vi "FipsAdjacent.vi"() -> (11 "Fips":i32[](array[numeric]))   [LabVIEW 2017] (continued)
VA\"\t51095\n\"New Kent County, VA\"\t51127\t\"King and Queen County, VA\"\t51097\n\"New Kent County, VA\"\t51127\t\"King William County, VA\"\t51101\n\"New Kent County, VA\"\t51127\t\"New Kent County, VA\"\t51127\n\"Northampton County, VA\"\t51131\t\"Accomack County, VA\"\t51001\n\"Northampton County, VA\"\t51131\t\"Mathews County, VA\"\t51115\n\"Northampton County, VA\"\t51131\t\"Middlesex County, VA\"\t51119\n\"Northampton County, VA\"\t51131\t\"Northampton County, VA\"\t51131\n\"Northampton County, VA\"\t51131\t\"York County, VA\"\t51199\n\"Northampton County, VA\"\t51131\t\"Hampton city, VA\"\t51650\n\"Northampton County, VA\"\t51131\t\"Norfolk city, VA\"\t51710\n\"Northampton County, VA\"\t51131\t\"Poquoson city, VA\"\t51735\n\"Northampton County, VA\"\t51131\t\"Virginia Beach city, VA\"\t51810\n\"Northumberland County, VA\"\t51133\t\"St. Mary's County, MD\"\t24037\n\"Northumberland County, VA\"\t51133\t\"Somerset County, MD\"\t24039\n\"Northumberland County, VA\"\t51133\t\"Accomack County, VA\"\t51001\n\"Northumberland County, VA\"\t51133\t\"Lancaster County, VA\"\t51103\n\"Northumberland County, VA\"\t51133\t\"Northumberland County, VA\"\t51133\n\"Northumberland County, VA\"\t51133\t\"Richmond County, VA\"\t51159\n\"Northumberland County, VA\"\t51133\t\"Westmoreland County, VA\"\t51193\n\"Nottoway County, VA\"\t51135\t\"Amelia County, VA\"\t51007\n\"Nottoway County, VA\"\t51135\t\"Brunswick County, VA\"\t51025\n\"Nottoway County, VA\"\t51135\t\"Dinwiddie County, VA\"\t51053\n\"Nottoway County, VA\"\t51135\t\"Lunenburg County, VA\"\t51111\n\"Nottoway County, VA\"\t51135\t\"Nottoway County, VA\"\t51135\n\"Nottoway County, VA\"\t51135\t\"Prince Edward County, VA\"\t51147\n\"Orange County, VA\"\t51137\t\"Albemarle County, VA\"\t51003\n\"Orange County, VA\"\t51137\t\"Culpeper County, VA\"\t51047\n\"Orange County, VA\"\t51137\t\"Greene County, VA\"\t51079\n\"Orange County, VA\"\t51137\t\"Louisa County, VA\"\t51109\n\"Orange County, VA\"\t51137\t\"Madison County, VA\"\t51113\n\"Orange County, VA\"\t51137\t\"Orange County, VA\"\t51137\n\"Orange County, VA\"\t51137\t\"Spotsylvania County, VA\"\t51177\n\"Page County, VA\"\t51139\t\"Greene County, VA\"\t51079\n\"Page County, VA\"\t51139\t\"Madison County, VA\"\t51113\n\"Page County, VA\"\t51139\t\"Page County, VA\"\t51139\n\"Page County, VA\"\t51139\t\"Rappahannock County, VA\"\t51157\n\"Page County, VA\"\t51139\t\"Rockingham County, VA\"\t51165\n\"Page County, VA\"\t51139\t\"Shenandoah County, VA\"\t51171\n\"Page County, VA\"\t51139\t\"Warren County, VA\"\t51187\n\"Patrick County, VA\"\t51141\t\"Stokes County, NC\"\t37169\n\"Patrick County, VA\"\t51141\t\"Surry County, NC\"\t37171\n\"Patrick County, VA\"\t51141\t\"Carroll County, VA\"\t51035\n\"Patrick County, VA\"\t51141\t\"Floyd County, VA\"\t51063\n\"Patrick County, VA\"\t51141\t\"Franklin County, VA\"\t51067\n\"Patrick County, VA\"\t51141\t\"Henry County, VA\"\t51089\n\"Patrick County, VA\"\t51141\t\"Patrick County, VA\"\t51141\n\"Pittsylvania County, VA\"\t51143\t\"Caswell County, NC\"\t37033\n\"Pittsylvania County, VA\"\t51143\t\"Rockingham County, NC\"\t37157\n\"Pittsylvania County, VA\"\t51143\t\"Bedford County, VA\"\t51019\n\"Pittsylvania County, VA\"\t51143\t\"Campbell County, VA\"\t51031\n\"Pittsylvania County, VA\"\t51143\t\"Franklin County, VA\"\t51067\n\"Pittsylvania County, VA\"\t51143\t\"Halifax County, VA\"\t51083\n\"Pittsylvania County, VA\"\t51143\t\"Henry County, VA\"\t51089\n\"Pittsylvania County, VA\"\t51143\t\"Pittsylvania County, VA\"\t51143\n\"Pittsylvania County, VA\"\t51143\t\"Danville city, VA\"\t51590\n\"Powhatan County, VA\"\t51145\t\"Amelia County, VA\"\t51007\n\"Powhatan County, VA\"\t51145\t\"Chesterfield County, VA\"\t51041\n\"Powhatan County, VA\"\t51145\t\"Cumberland County, VA\"\t51049\n\"Powhatan County, VA\"\t51145\t\"Goochland County, VA\"\t51075\n\"Powhatan County, VA\"\t51145\t\"Henrico County, VA\"\t51087\n\"Powhatan County, VA\"\t51145\t\"Powhatan County, VA\"\t51145\n\"Prince Edward County, VA\"\t51147\t\"Amelia County, VA\"\t51007\n\"Prince Edward County, VA\"\t51147\t\"Appomattox County, VA\"\t51011\n\"Prince Edward County, VA\"\t51147\t\"Buckingham County, VA\"\t51029\n\"Prince Edward County, VA\"\t51147\t\"Charlotte County, VA\"\t51037\n\"Prince Edward County, VA\"\t51147\t\"Cumberland County, VA\"\t51049\n\"Prince Edward County, VA\"\t51147\t\"Lunenburg County, VA\"\t51111\n\"Prince Edward County, VA\"\t51147\t\"Nottoway County, VA\"\t51135\n\"Prince Edward County, VA\"\t51147\t\"Prince Edward County, VA\"\t51147\n\"Prince George County, VA\"\t51149\t\"Charles City County, VA\"\t51036\n\"Prince George County, VA\"\t51149\t\"Chesterfield County, VA\"\t51041\n\"Prince George County, VA\"\t51149\t\"Dinwiddie County, VA\"\t51053\n\"Prince George County, VA\"\t51149\t\"Prince George County, VA\"\t51149\n\"Prince George County, VA\"\t51149\t\"Surry County, VA\"\t51181\n\"Prince George County, VA\"\t51149\t\"Sussex County, VA\"\t51183\n\"Prince George County, VA\"\t51149\t\"Hopewell city, VA\"\t51670\n\"Prince George County, VA\"\t51149\t\"Petersburg city, VA\"\t51730\n\"Prince William County, VA\"\t51153\t\"Charles County, MD\"\t24017\n\"Prince William County, VA\"\t51153\t\"Fairfax County, VA\"\t51059\n\"Prince William County, VA\"\t51153\t\"Fauquier County, VA\"\t51061\n\"Prince William County, VA\"\t51153\t\"Loudoun County, VA\"\t51107\n\"Prince William County, VA\"\t51153\t\"Prince William County, VA\"\t51153\n\"Prince William County, VA\"\t51153\t\"Stafford County, VA\"\t51179\n\"Prince William County, VA\"\t51153\t\"Manassas city, VA\"\t51683\n\"Prince William County, VA\"\t51153\t\"Manassas Park city, VA\"\t51685\n\"Pulaski County, VA\"\t51155\t\"Bland County, VA\"\t51021\n\"Pulaski County, VA\"\t51155\t\"Carroll County, VA\"\t51035\n\"Pulaski County, VA\"\t51155\t\"Floyd County, VA\"\t51063\n\"Pulaski County, VA\"\t51155\t\"Giles County, VA\"\t51071\n\"Pulaski County, VA\"\t51155\t\"Montgomery County, VA\"\t51121\n\"Pulaski County, VA\"\t51155\t\"Pulaski County, VA\"\t51155\n\"Pulaski County, VA\"\t51155\t\"Wythe County, VA\"\t51197\n\"Pulaski County, VA\"\t51155\t\"Radford city, VA\"\t51750\n\"Rappahannock County, VA\"\t51157\t\"Culpeper County, VA\"\t51047\n\"Rappahannock County, VA\"\t51157\t\"Fauquier County, VA\"\t51061\n\"Rappahannock County, VA\"\t51157\t\"Madison County, VA\"\t51113\n\"Rappahannock County, VA\"\t51157\t\"Page County, VA\"\t51139\n\"Rappahannock County, VA\"\t51157\t\"Rappahannock County, VA\"\t51157\n\"Rappahannock County, VA\"\t51157\t\"Warren County, VA\"\t51187\n\"Richmond County, VA\"\t51159\t\"Essex County, VA\"\t51057\n\"Richmond County, VA\"\t51159\t\"Lancaster County, VA\"\t51103\n\"Richmond County, VA\"\t51159\t\"Middlesex County, VA\"\t51119\n\"Richmond County, VA\"\t51159\t\"Northumberland County, VA\"\t51133\n\"Richmond County, VA\"\t51159\t\"Richmond County, VA\"\t51159\n\"Richmond County, VA\"\t51159\t\"Westmoreland County, VA\"\t51193\n\"Roanoke County, VA\"\t51161\t\"Bedford County, VA\"\t51019\n\"Roanoke County, VA\"\t51161\t\"Botetourt County, VA\"\t51023\n\"Roanoke County, VA\"\t51161\t\"Craig County, VA\"\t51045\n\"Roanoke County, VA\"\t51161\t\"Floyd County, VA\"\t51063\n\"Roanoke County, VA\"\t51161\t\"Franklin County, VA\"\t51067\n\"Roanoke County, VA\"\t51161\t\"Montgomery County, VA\"\t51121\n\"Roanoke County, VA\"\t51161\t\"Roanoke County, VA\"\t51161\n\"Roanoke County, VA\"\t51161\t\"Roanoke city, VA\"\t51770\n\"Roanoke County, VA\"\t51161\t\"Salem city, VA\"\t51775\n\"Rockbridge County, VA\"\t51163\t\"Alleghany County, VA\"\t51005\n\"Rockbridge County, VA\"\t51163\t\"Amherst County, VA\"\t51009\n\"Rockbridge County, VA\"\t51163\t\"Augusta County, VA\"\t51015\n\"Rockbridge County, VA\"\t51163\t\"Bath County, VA\"\t51017\n\"Rockbridge County, VA\"\t51163\t\"Bedford County, VA\"\t51019\n\"Rockbridge County, VA\"\t51163\t\"Botetourt County, VA\"\t51023\n\"Rockbridge County, VA\"\t51163\t\"Nelson County, VA\"\t51125\n\"Rockbridge County, VA\"\t51163\t\"Rockbridge County, VA\"\t51163\n\"Rockbridge County, VA\"\t51163\t\"Buena Vista city, VA\"\t51530\n\"Rockbridge County, VA\"\t51163\t\"Lexington city, VA\"\t51678\n\"Rockingham County, VA\"\t51165\t\"Albemarle County, VA\"\t51003\n\"Rockingham County, VA\"\t51165\t\"Augusta County, VA\"\t51015\n\"Rockingham County, VA\"\t51165\t\"Greene County, VA\"\t51079\n\"Rockingham County, VA\"\t51165\t\"Page County, VA\"\t51139\n\"Rockingham County, VA\"\t51165\t\"Rockingham County, VA\"\t51165\n\"Rockingham County, VA\"\t51165\t\"Shenandoah County, VA\"\t51171\n\"Rockingham County, VA\"\t51165\t\"Harrisonburg city, VA\"\t51660\n\"Rockingham County, VA\"\t51165\t\"Hardy County, WV\"\t54031\n\"Rockingham County, VA\"\t51165\t\"Pendleton County, WV\"\t54071\n\"Russell County, VA\"\t51167\t\"Buchanan County, VA\"\t51027\n\"Russell County, VA\"\t51167\t\"Dickenson County, VA\"\t51051\n\"Russell County, VA\"\t51167\t\"Russell County, VA\"\t51167\n\"Russell County, VA\"\t51167\t\"Scott County, VA\"\t51169\n\"Russell County, VA\"\t51167\t\"Smyth County, VA\"\t51173\n\"Russell County, VA\"\t51167\t\"Tazewell County, VA\"\t51185\n\"Russell County, VA\"\t51167\t\"Washington County, VA\"\t51191\n\"Russell County, VA\"\t51167\t\"Wise County, VA\"\t51195\n\"Scott County, VA\"\t51169\t\"Hancock County, TN\"\t47067\n\"Scott County, VA\"\t51169\t\"Hawkins County, TN\"\t47073\n\"Scott County, VA\"\t51169\t\"Sullivan County, TN\"\t47163\n\"Scott County, VA\"\t51169\t\"Lee County, VA\"\t51105\n\"Scott County, VA\"\t51169\t\"Russell County, VA\"\t51167\n\"Scott County, VA\"\t51169\t\"Scott County, VA\"\t51169\n\"Scott County, VA\"\t51169\t\"Washington County, VA\"\t51191\n\"Scott County, VA\"\t51169\t\"Wise County, VA\"\t51195\n\"Shenandoah County, VA\"\t51171\t\"Frederick County, VA\"\t51069\n\"Shenandoah County, VA\"\t51171\t\"Page County, VA\"\t51139\n\"Shenandoah County, VA\"\t51171\t\"Rockingham County, VA\"\t51165\n\"Shenandoah County, VA\"\t51171\t\"Shenandoah County, VA\"\t51171\n\"Shenandoah County, VA\"\t51171\t\"Warren County, VA\"\t51187\n\"Shenandoah County, VA\"\t51171\t\"Hardy County, WV\"\t54031\n\"Smyth County, VA\"\t51173\t\"Bland County, VA\"\t51021\n\"Smyth County, VA\"\t51173\t\"Grayson County, VA\"\t51077\n\"Smyth County, VA\"\t51173\t\"Russell County, VA\"\t51167\n\"Smyth County, VA\"\t51173\t\"Smyth County, VA\"\t51173\n\"Smyth County, VA\"\t51173\t\"Tazewell County, VA\"\t51185\n\"Smyth County, VA\"\t51173\t\"Washington County, VA\"\t51191\n\"Smyth County, VA\"\t51173\t\"Wythe County, VA\"\t51197\n\"Southampton County, VA\"\t51175\t\"Gates County, NC\"\t37073\n\"Southampton County, VA\"\t51175\t\"Hertford County, NC\"\t37091\n\"Southampton County, VA\"\t51175\t\"Northampton County, NC\"\t37131\n\"Southampton County, VA\"\t51175\t\"Greensville County, VA\"\t51081\n\"Southampton County, VA\"\t51175\t\"Isle of Wight County, VA\"\t51093\n\"Southampton County, VA\"\t51175\t\"Southampton County, VA\"\t51175\n\"Southampton County, VA\"\t51175\t\"Surry County, VA\"\t51181\n\"Southampton County, VA\"\t51175\t\"Sussex County, VA\"\t51183\n\"Southampton County, VA\"\t51175\t\"Franklin city, VA\"\t51620\n\"Southampton County, VA\"\t51175\t\"Suffolk city, VA\"\t51800\n\"Spotsylvania County, VA\"\t51177\t\"Caroline County, VA\"\t51033\n\"Spotsylvania County, VA\"\t51177\t\"Culpeper County, VA\"\t51047\n\"Spotsylvania County, VA\"\t51177\t\"Hanover County, VA\"\t51085\n\"Spotsylvania County, VA\"\t51177\t\"Louisa County, VA\"\t51109\n\"Spotsylvania County, VA\"\t51177\t\"Orange County, VA\"\t51137\n\"Spotsylvania County, VA\"\t51177\t\"Spotsylvania County, VA\"\t51177\n\"Spotsylvania County, VA\"\t51177\t\"Stafford County, VA\"\t51179\n\"Spotsylvania County, VA\"\t51177\t\"Fredericksburg city, VA\"\t51630\n\"Stafford County, VA\"\t51179\t\"Charles County, MD\"\t24017\n\"Stafford County, VA\"\t51179\t\"Caroline County, VA\"\t51033\n\"Stafford County, VA\"\t51179\t\"Culpeper County, VA\"\t51047\n\"Stafford County, VA\"\t51179\t\"Fauquier County, VA\"\t51061\n\"Stafford County, VA\"\t51179\t\"King George County, VA\"\t51099\n\"Stafford County, VA\"\t51179\t\"Prince William County, VA\"\t51153\n\"Stafford County, VA\"\t51179\t\"Spotsylvania County, VA\"\t51177\n\"Stafford County, VA\"\t51179\t\"Stafford County, VA\"\t51179\n\"Stafford County, VA\"\t51179\t\"Fredericksburg city, VA\"\t51630\n\"Surry County, VA\"\t51181\t\"Charles City County, VA\"\t51036\n\"Surry County, VA\"\t51181\t\"Isle of Wight County, VA\"\t51093\n\"Surry County, VA\"\t51181\t\"James City County, VA\"\t51095\n\"Surry County, VA\"\t51181\t\"Prince George County, VA\"\t51149\n\"Surry County, VA\"\t51181\t\"Southampton County, VA\"\t51175\n\"Surry County, VA\"\t51181\t\"Surry County, VA\"\t51181\n\"Surry County, VA\"\t51181\t\"Sussex County, VA\"\t51183\n\"Surry County, VA\"\t51181\t\"Newport News city, VA\"\t51700\n\"Sussex County, VA\"\t51183\t\"Dinwiddie County, VA\"\t51053\n\"Sussex County, VA\"\t51183\t\"Greensville County, VA\"\t51081\n\"Sussex County, VA\"\t51183\t\"Prince George County, VA\"\t51149\n\"Sussex County, VA\"\t51183\t\"Southampton County, VA\"\t51175\n\"Sussex County, VA\"\t51183\t\"Surry County, VA\"\t51181\n\"Sussex County, VA\"\t51183\t\"Sussex County, VA\"\t51183\n\"Tazewell County, VA\"\t51185\t\"Bland County, VA\"\t51021\n\"Tazewell County, VA\"\t51185\t\"Buchanan County, VA\"\t51027\n\"Tazewell County, VA\"\t51185\t\"Russell County, VA\"\t51167\n\"Tazewell County, VA\"\t51185\t\"Smyth County, VA\"\t51173\n\"Tazewell County, VA\"\t51185\t\"Tazewell County, VA\"\t51185\n\"Tazewell County, VA\"\t51185\t\"McDowell County, WV\"\t54047\n\"Tazewell County, VA\"\t51185\t\"Mercer County, WV\"\t54055\n\"Warren County, VA\"\t51187\t\"Clarke County, VA\"\t51043\n\"Warren County, VA\"\t51187\t\"Fauquier County, VA\"\t51061\n\"Warren County, VA\"\t51187\t\"Frederick County, VA\"\t51069\n\"Warren County, VA\"\t51187\t\"Page County, VA\"\t51139\n\"Warren County, VA\"\t51187\t\"Rappahannock County, VA\"\t51157\n\"Warren County, VA\"\t51187\t\"Shenandoah County, VA\"\t51171\n\"Warren County, VA\"\t51187\t\"Warren County, VA\"\t51187\n\"Washington County, VA\"\t51191\t\"Johnson County, TN\"\t47091\n\"Washington County, VA\"\t51191\t\"Sullivan County, TN\"\t47163\n\"Washington County, VA\"\t51191\t\"Grayson County, VA\"\t51077\n\"Washington County, VA\"\t51191\t\"Russell County, VA\"\t51167\n\"Washington County, VA\"\t51191\t\"Scott County, VA\"\t51169\n\"Washington County, VA\"\t51191\t\"Smyth County, VA\"\t51173\n\"Washington County, VA\"\t51191\t\"Washington County, VA\"\t51191\n\"Washington County, VA\"\t51191\t\"Bristol city, VA\"\t51520\n\"Westmoreland County, VA\"\t51193\t\"Charles County, MD\"\t24017\n\"Westmoreland County, VA\"\t51193\t\"St. Mary's County, MD\"\t24037\n\"Westmoreland County, VA\"\t51193\t\"Essex County, VA\"\t51057\n\"Westmoreland County, VA\"\t51193\t\"King George County, VA\"\t51099\n\"Westmoreland County, VA\"\t51193\t\"Northumberland County, VA\"\t51133\n\"Westmoreland County, VA\"\t51193\t\"Richmond County, VA\"\t51159\n\"Westmoreland County, VA\"\t51193\t\"Westmoreland County, VA\"\t51193\n\"Wise County, VA\"\t51195\t\"Harlan County, KY\"\t21095\n\"Wise County, VA\"\t51195\t\"Letcher County, KY\"\t21133\n\"Wise County, VA\"\t51195\t\"Pike County, KY\"\t21195\n\"Wise County, VA\"\t51195\t\"Dickenson County, VA\"\t51051\n\"Wise County, VA\"\t51195\t\"Lee County, VA\"\t51105\n\"Wise County, VA\"\t51195\t\"Russell County, VA\"\t51167\n\"Wise County, VA\"\t51195\t\"Scott County, VA\"\t51169\n\"Wise County, VA\"\t51195\t\"Wise County, VA\"\t51195\n\"Wise County, VA\"\t51195\t\"Norton city, VA\"\t51720\n\"Wythe County, VA\"\t51197\t\"Bland County, VA\"\t51021\n\"Wythe County, VA\"\t51197\t\"Carroll County, VA\"\t51035\n\"Wythe County, VA\"\t51197\t\"Grayson County, VA\"\t51077\n\"Wythe County, VA\"\t51197\t\"Pulaski County, VA\"\t51155\n\"Wythe County, VA\"\t51197\t\"Smyth County, VA\"\t51173\n\"Wythe County, VA\"\t51197\t\"Wythe County, VA\"\t51197\n\"York County, VA\"\t51199\t\"Gloucester County, VA\"\t51073\n\"York County, VA\"\t51199\t\"James City County, VA\"\t51095\n\"York County, VA\"\t51199\t\"Mathews County, VA\"\t51115\n\"York County, VA\"\t51199\t\"Northampton County, VA\"\t51131\n\"York County, VA\"\t51199\t\"York County, VA\"\t51199\n\"York County, VA\"\t51199\t\"Hampton city, VA\"\t51650\n\"York County, VA\"\t51199\t\"Newport News city, VA\"\t51700\n\"York County, VA\"\t51199\t\"Poquoson city, VA\"\t51735\n\"York County, VA\"\t51199\t\"Williamsburg city, VA\"\t51830\n\"Alexandria city, VA\"\t51510\t\"District of Columbia, DC\"\t11001\n\"Alexandria city, VA\"\t51510\t\"Prince George's County, MD\"\t24033\n\"Alexandria city, VA\"\t51510\t\"Arlington County, VA\"\t51013\n\"Alexandria city, VA\"\t51510\t\"Fairfax County, VA\"\t51059\n\"Alexandria city, VA\"\t51510\t\"Alexandria city, VA\"\t51510\n\"Bedford city, VA\"\t51515\t\"Bedford County, VA\"\t51019\n\"Bedford city, VA\"\t51515\t\"Bedford city, VA\"\t51515\n\"Bristol city, VA\"\t51520\t\"Sullivan County, TN\"\t47163\n\"Bristol city, VA\"\t51520\t\"Washington County, VA\"\t51191\n\"Bristol city, VA\"\t51520\t\"Bristol city, VA\"\t51520\n\"Buena Vista city, VA\"\t51530\t\"Rockbridge County, VA\"\t51163\n\"Buena Vista city, VA\"\t51530\t\"Buena Vista city, VA\"\t51530\n\"Charlottesville city, VA\"\t51540\t\"Albemarle County, VA\"\t51003\n\"Charlottesville city, VA\"\t51540\t\"Charlottesville city, VA\"\t51540\n\"Chesapeake city, VA\"\t51550\t\"Camden County, NC\"\t37029\n\"Chesapeake city, VA\"\t51550\t\"Currituck County, NC\"\t37053\n\"Chesapeake city, VA\"\t51550\t\"Chesapeake city, VA\"\t51550\n\"Chesapeake city, VA\"\t51550\t\"Norfolk city, VA\"\t51710\n\"Chesapeake city, VA\"\t51550\t\"Portsmouth city, VA\"\t51740\n\"Chesapeake city, VA\"\t51550\t\"Suffolk city, VA\"\t51800\n\"Chesapeake city, VA\"\t51550\t\"Virginia Beach city, VA\"\t51810\n\"Colonial Heights city, VA\"\t51570\t\"Chesterfield County, VA\"\t51041\n\"Colonial Heights city, VA\"\t51570\t\"Colonial Heights city, VA\"\t51570\n\"Colonial Heights city, VA\"\t51570\t\"Petersburg city, VA\"\t51730\n\"Covington city, VA\"\t51580\t\"Alleghany County, VA\"\t51005\n\"Covington city, VA\"\t51580\t\"Covington city, VA\"\t51580\n\"Danville city, VA\"\t51590\t\"Caswell County, NC\"\t37033\n\"Danville city, VA\"\t51590\t\"Pittsylvania County, VA\"\t51143\n\"Danville city, VA\"\t51590\t\"Danville city, VA\"\t51590\n\"Emporia city, VA\"\t51595\t\"Greensville County, VA\"\t51081\n\"Emporia city, VA\"\t51595\t\"Emporia city, VA\"\t51595\n\"Fairfax city, VA\"\t51600\t\"Fairfax County, VA\"\t51059\n\"Fairfax city, VA\"\t51600\t\"Fairfax city, VA\"\t51600\n\"Falls Church city, VA\"\t51610\t\"Arlington County, VA\"\t51013\n\"Falls Church city, VA\"\t51610\t\"Fairfax County, VA\"\t51059\n\"Falls Church city, VA\"\t51610\t\"Falls Church city, VA\"\t51610\n\"Franklin city, VA\"\t51620\t\"Isle of Wight County, VA\"\t51093\n\"Franklin city, VA\"\t51620\t\"Southampton County, VA\"\t51175\n\"Franklin city, VA\"\t51620\t\"Franklin city, VA\"\t51620\n\"Fredericksburg city, VA\"\t51630\t\"Spotsylvania County, VA\"\t51177\n\"Fredericksburg city, VA\"\t51630\t\"Stafford County, VA\"\t51179\n\"Fredericksburg city, VA\"\t51630\t\"Fredericksburg city, VA\"\t51630\n\"Galax city, VA\"\t51640\t\"Carroll County, VA\"\t51035\n\"Galax city, VA\"\t51640\t\"Grayson County, VA\"\t51077\n\"Galax city, VA\"\t51640\t\"Galax city, VA\"\t51640\n\"Hampton city, VA\"\t51650\t\"Northampton County, VA\"\t51131\n\"Hampton city, VA\"\t51650\t\"York County, VA\"\t51199\n\"Hampton city, VA\"\t51650\t\"Hampton city, VA\"\t51650\n\"Hampton city, VA\"\t51650\t\"Newport News city, VA\"\t51700\n\"Hampton city, VA\"\t51650\t\"Norfolk city, VA\"\t51710\n\"Hampton city, VA\"\t51650\t\"Poquoson city, VA\"\t51735\n\"Hampton city, VA\"\t51650\t\"Portsmouth city, VA\"\t51740\n\"Hampton city, VA\"\t51650\t\"Virginia Beach city, VA\"\t51810\n\"Harrisonburg city, VA\"\t51660\t\"Rockingham County, VA\"\t51165\n\"Harrisonburg city, VA\"\t51660\t\"Harrisonburg city, VA\"\t51660\n\"Hopewell city, VA\"\t51670\t\"Chesterfield County, VA\"\t51041\n\"Hopewell city, VA\"\t51670\t\"Prince George County, VA\"\t51149\n\"Hopewell city, VA\"\t51670\t\"Hopewell city, VA\"\t51670\n\"Lexington city, VA\"\t51678\t\"Rockbridge County, VA\"\t51163\n\"Lexington city, VA\"\t51678\t\"Lexington city, VA\"\t51678\n\"Lynchburg city, VA\"\t51680\t\"Amherst County, VA\"\t51009\n\"Lynchburg city, VA\"\t51680\t\"Bedford County, VA\"\t51019\n\"Lynchburg city, VA\"\t51680\t\"Campbell County, VA\"\t51031\n\"Lynchburg city, VA\"\t51680\t\"Lynchburg city, VA\"\t51680\n\"Manassas city, VA\"\t51683\t\"Prince William County, VA\"\t51153\n\"Manassas city, VA\"\t51683\t\"Manassas city, VA\"\t51683\n\"Manassas city, VA\"\t51683\t\"Manassas Park city, VA\"\t51685\n\"Manassas Park city, VA\"\t51685\t\"Prince William County, VA\"\t51153\n\"Manassas Park city, VA\"\t51685\t\"Manassas city, VA\"\t51683\n\"Manassas Park city, VA\"\t51685\t\"Manassas Park city, VA\"\t51685\n\"Martinsville city, VA\"\t51690\t\"Henry County, VA\"\t51089\n\"Martinsville city, VA\"\t51690\t\"Martinsville city, VA\"\t51690\n\"Newport News city, VA\"\t51700\t\"Isle of Wight County, VA\"\t51093\n\"Newport News city, VA\"\t51700\t\"James City County, VA\"\t51095\n\"Newport News city, VA\"\t51700\t\"Surry County, VA\"\t51181\n\"Newport News city, VA\"\t51700\t\"York County, VA\"\t51199\n\"Newport News city, VA\"\t51700\t\"Hampton city, VA\"\t51650\n\"Newport News city, VA\"\t51700\t\"Newport News city, VA\"\t51700\n\"Newport News city, VA\"\t51700\t\"Portsmouth city, VA\"\t51740\n\"Newport News city, VA\"\t51700\t\"Suffolk city, VA\"\t51800\n\"Norfolk city, VA\"\t51710\t\"Northampton County, VA\"\t51131\n\"Norfolk city, VA\"\t51710\t\"Chesapeake city, VA\"\t51550\n\"Norfolk city, VA\"\t51710\t\"Hampton city, VA\"\t51650\n\"Norfolk city, VA\"\t51710\t\"Norfolk city, VA\"\t51710\n\"Norfolk city, VA\"\t51710\t\"Portsmouth city, VA\"\t51740\n\"Norfolk city, VA\"\t51710\t\"Virginia Beach city, VA\"\t51810\n\"Norton city, VA\"\t51720\t\"Wise County, VA\"\t51195\n\"Norton city, VA\"\t51720\t\"Norton city, VA\"\t51720\n\"Petersburg city, VA\"\t51730\t\"Chesterfield County, VA\"\t51041\n\"Petersburg city, VA\"\t51730\t\"Dinwiddie County, VA\"\t51053\n\"Petersburg city, VA\"\t51730\t\"Prince George County, VA\"\t51149\n\"Petersburg city, VA\"\t51730\t\"Colonial Heights city, VA\"\t51570\n\"Petersburg city, VA\"\t51730\t\"Petersburg city, VA\"\t51730\n\"Poquoson city, VA\"\t51735\t\"Northampton County, VA\"\t51131\n\"Poquoson city, VA\"\t51735\t\"York County, VA\"\t51199\n\"Poquoson city, VA\"\t51735\t\"Hampton city, VA\"\t51650\n\"Poquoson city, VA\"\t51735\t\"Poquoson city, VA\"\t51735\n\"Portsmouth city, VA\"\t51740\t\"Chesapeake city, VA\"\t51550\n\"Portsmouth city, VA\"\t51740\t\"Hampton city, VA\"\t51650\n\"Portsmouth city, VA\"\t51740\t\"Newport News city, VA\"\t51700\n\"Portsmouth city, VA\"\t51740\t\"Norfolk city, VA\"\t51710\n\"Portsmouth city, VA\"\t51740\t\"Portsmouth city, VA\"\t51740\n\"Portsmouth city, VA\"\t51740\t\"Suffolk city, VA\"\t51800\n\"Radford city, VA\"\t51750\t\"Montgomery County, VA\"\t51121\n\"Radford city, VA\"\t51750\t\"Pulaski County, VA\"\t51155\n\"Radford city, VA\"\t51750\t\"Radford city, VA\"\t51750\n\"Richmond city, VA\"\t51760\t\"Chesterfield County, VA\"\t51041\n\"Richmond city, VA\"\t51760\t\"Henrico County, VA\"\t51087\n\"Richmond city, VA\"\t51760\t\"Richmond city, VA\"\t51760\n\"Roanoke city, VA\"\t51770\t\"Roanoke County, VA\"\t51161\n\"Roanoke city, VA\"\t51770\t\"Roanoke city, VA\"\t51770\n\"Roanoke city, VA\"\t51770\t\"Salem city, VA\"\t51775\n\"Salem city, VA\"\t51775\t\"Roanoke County, VA\"\t51161\n\"Salem city, VA\"\t51775\t\"Roanoke city, VA\"\t51770\n\"Salem city, VA\"\t51775\t\"Salem city, VA\"\t51775\n\"Staunton city, VA\"\t51790\t\"Augusta County, VA\"\t51015\n\"Staunton city, VA\"\t51790\t\"Staunton city, VA\"\t51790\n\"Suffolk city, VA\"\t51800\t\"Camden County, NC\"\t37029\n\"Suffolk city, VA\"\t51800\t\"Gates County, NC\"\t37073\n\"Suffolk city, VA\"\t51800\t\"Isle of Wight County, VA\"\t51093\n\"Suffolk city, VA\"\t51800\t\"Southampton County, VA\"\t51175\n\"Suffolk city, VA\"\t51800\t\"Chesapeake city, VA\"\t51550\n\"Suffolk city, VA\"\t51800\t\"Newport News city, VA\"\t51700\n\"Suffolk city, VA\"\t51800\t\"Portsmouth city, VA\"\t51740\n\"Suffolk city, VA\"\t51800\t\"Suffolk city, VA\"\t51800\n\"Virginia Beach city, VA\"\t51810\t\"Currituck County, NC\"\t37053\n\"Virginia Beach city, VA\"\t51810\t\"Northampton County, VA\"\t51131\n\"Virginia Beach city, VA\"\t51810\t\"Chesapeake city, VA\"\t51550\n\"Virginia Beach city, VA\"\t51810\t\"Hampton city, VA\"\t51650\n\"Virginia Beach city, VA\"\t51810\t\"Norfolk city, VA\"\t51710\n\"Virginia Beach city, VA\"\t51810\t\"Virginia Beach city, VA\"\t51810\n\"Waynesboro city, VA\"\t51820\t\"Augusta County, VA\"\t51015\n\"Waynesboro city, VA\"\t51820\t\"Waynesboro city, VA\"\t51820\n\"Williamsburg city, VA\"\t51830\t\"James City County, VA\"\t51095\n\"Williamsburg city, VA\"\t51830\t\"York County, VA\"\t51199\n\"Williamsburg city, VA\"\t51830\t\"Williamsburg city, VA\"\t51830\n\"Winchester city, VA\"\t51840\t\"Frederick County, VA\"\t51069\n\"Winchester city, VA\"\t51840\t\"Winchester city, VA\"\t51840\n\"Adams County, WA\"\t53001\t\"Adams County, WA\"\t53001\n\"Adams County, WA\"\t53001\t\"Franklin County, WA\"\t53021\n\"Adams County, WA\"\t53001\t\"Grant County, WA\"\t53025\n\"Adams County, WA\"\t53001\t\"Lincoln County, WA\"\t53043\n\"Adams County, WA\"\t53001\t\"Whitman County, WA\"\t53075\n\"Asotin County, WA\"\t53003\t\"Nez Perce County, ID\"\t16069\n\"Asotin County, WA\"\t53003\t\"Wallowa County, OR\"\t41063\n\"Asotin County, WA\"\t53003\t\"Asotin County, WA\"\t53003\n\"Asotin County, WA\"\t53003\t\"Garfield County, WA\"\t53023\n\"Asotin County, WA\"\t53003\t\"Whitman County, WA\"\t53075\n\"Benton County, WA\"\t53005\t\"Morrow County, OR\"\t41049\n\"Benton County, WA\"\t53005\t\"Umatilla County, OR\"\t41059\n\"Benton County, WA\"\t53005\t\"Benton County, WA\"\t53005\n\"Benton County, WA\"\t53005\t\"Franklin County, WA\"\t53021\n\"Benton County, WA\"\t53005\t\"Grant County, WA\"\t53025\n\"Benton County, WA\"\t53005\t\"Klickitat County, WA\"\t53039\n\"Benton County, WA\"\t53005\t\"Walla Walla County, WA\"\t53071\n\"Benton County, WA\"\t53005\t\"Yakima County, WA\"\t53077\n\"Chelan County, WA\"\t53007\t\"Chelan County, WA\"\t53007\n\"Chelan County, WA\"\t53007\t\"Douglas County, WA\"\t53017\n\"Chelan County, WA\"\t53007\t\"King County, WA\"\t53033\n\"Chelan County, WA\"\t53007\t\"Kittitas County, WA\"\t53037\n\"Chelan County, WA\"\t53007\t\"Okanogan County, WA\"\t53047\n\"Chelan County, WA\"\t53007\t\"Skagit County, WA\"\t53057\n\"Chelan County, WA\"\t53007\t\"Snohomish County, WA\"\t53061\n\"Clallam County, WA\"\t53009\t\"Clallam County, WA\"\t53009\n\"Clallam County, WA\"\t53009\t\"Jefferson County, WA\"\t53031\n\"Clallam County, WA\"\t53009\t\"San Juan County, WA\"\t53055\n\"Clark County, WA\"\t53011\t\"Columbia County, OR\"\t41009\n\"Clark County, WA\"\t53011\t\"Multnomah County, OR\"\t41051\n\"Clark County, WA\"\t53011\t\"Clark County, WA\"\t53011\n\"Clark County, WA\"\t53011\t\"Cowlitz County, WA\"\t53015\n\"Clark County, WA\"\t53011\t\"Skamania County, WA\"\t53059\n\"Columbia County, WA\"\t53013\t\"Umatilla County, OR\"\t41059\n\"Columbia County, WA\"\t53013\t\"Wallowa County, OR\"\t41063\n\"Columbia County, WA\"\t53013\t\"Columbia County, WA\"\t53013\n\"Columbia County, WA\"\t53013\t\"Franklin County, WA\"\t53021\n\"Columbia County, WA\"\t53013\t\"Garfield County, WA\"\t53023\n\"Columbia County, WA\"\t53013\t\"Walla Walla County, WA\"\t53071\n\"Columbia County, WA\"\t53013\t\"Whitman County, WA\"\t53075\n\"Cowlitz County, WA\"\t53015\t\"Columbia County, OR\"\t41009\n\"Cowlitz County, WA\"\t53015\t\"Clark County, WA\"\t53011\n\"Cowlitz County, WA\"\t53015\t\"Cowlitz County, WA\"\t53015\n\"Cowlitz County, WA\"\t53015\t\"Lewis County, WA\"\t53041\n\"Cowlitz County, WA\"\t53015\t\"Skamania County, WA\"\t53059\n\"Cowlitz County, WA\"\t53015\t\"Wahkiakum County, WA\"\t53069\n\"Douglas County, WA\"\t53017\t\"Chelan County, WA\"\t53007\n\"Douglas County, WA\"\t53017\t\"Douglas County, WA\"\t53017\n\"Douglas County, WA\"\t53017\t\"Grant County, WA\"\t53025\n\"Douglas County, WA\"\t53017\t\"Kittitas County, WA\"\t53037\n\"Douglas County, WA\"\t53017\t\"Okanogan County, WA\"\t53047\n\"Ferry County, WA\"\t53019\t\"Ferry County, WA\"\t53019\n\"Ferry County, WA\"\t53019\t\"Lincoln County, WA\"\t53043\n\"Ferry County, WA\"\t53019\t\"Okanogan County, WA\"\t53047\n\"Ferry County, WA\"\t53019\t\"Stevens County, WA\"\t53065\n\"Franklin County, WA\"\t53021\t\"Adams County, WA\"\t53001\n\"Franklin County, WA\"\t53021\t\"Benton County, WA\"\t53005\n\"Franklin County, WA\"\t53021\t\"Columbia County, WA\"\t53013\n\"Franklin County, WA\"\t53021\t\"Franklin County, WA\"\t53021\n\"Franklin County, WA\"\t53021\t\"Grant County, WA\"\t53025\n\"Franklin County, WA\"\t53021\t\"Walla Walla County, WA\"\t53071\n\"Franklin County, WA\"\t53021\t\"Whitman County, WA\"\t53075\n\"Garfield County, WA\"\t53023\t\"Wallowa County, OR\"\t41063\n\"Garfield County, WA\"\t53023\t\"Asotin County, WA\"\t53003\n\"Garfield County, WA\"\t53023\t\"Columbia County, WA\"\t53013\n\"Garfield County, WA\"\t53023\t\"Garfield County, WA\"\t53023\n\"Garfield County, WA\"\t53023\t\"Whitman County, WA\"\t53075\n\"Grant County, WA\"\t53025\t\"Adams County, WA\"\t53001\n\"Grant County, WA\"\t53025\t\"Benton County, WA\"\t53005\n\"Grant County, WA\"\t53025\t\"Douglas County, WA\"\t53017\n\"Grant County, WA\"\t53025\t\"Franklin County, WA\"\t53021\n\"Grant County, WA\"\t53025\t\"Grant County, WA\"\t53025\n\"Grant County, WA\"\t53025\t\"Kittitas County, WA\"\t53037\n\"Grant County, WA\"\t53025\t\"Lincoln County, WA\"\t53043\n\"Grant County, WA\"\t53025\t\"Okanogan County, WA\"\t53047\n\"Grant County, WA\"\t53025\t\"Yakima County, WA\"\t53077\n\"Grays Harbor County, WA\"\t53027\t\"Grays Harbor County, WA\"\t53027\n\"Grays Harbor County, WA\"\t53027\t\"Jefferson County, WA\"\t53031\n\"Grays Harbor County, WA\"\t53027\t\"Lewis County, WA\"\t53041\n\"Grays Harbor County, WA\"\t53027\t\"Mason County, WA\"\t53045\n\"Grays Harbor County, WA\"\t53027\t\"Pacific County, WA\"\t53049\n\"Grays Harbor County, WA\"\t53027\t\"Thurston County, WA\"\t53067\n\"Island County, WA\"\t53029\t\"Island County, WA\"\t53029\n\"Island County, WA\"\t53029\t\"Jefferson County, WA\"\t53031\n\"Island County, WA\"\t53029\t\"Kitsap County, WA\"\t53035\n\"Island County, WA\"\t53029\t\"San Juan County, WA\"\t53055\n\"Island County, WA\"\t53029\t\"Skagit County, WA\"\t53057\n\"Island County, WA\"\t53029\t\"Snohomish County, WA\"\t53061\n\"Jefferson County, WA\"\t53031\t\"Clallam County, WA\"\t53009\n\"Jefferson County, WA\"\t53031\t\"Grays Harbor County, WA\"\t53027\n\"Jefferson County, WA\"\t53031\t\"Island County, WA\"\t53029\n\"Jefferson County, WA\"\t53031\t\"Jefferson County, WA\"\t53031\n\"Jefferson County, WA\"\t53031\t\"Kitsap County, WA\"\t53035\n\"Jefferson County, WA\"\t53031\t\"Mason County, WA\"\t53045\n\"Jefferson County, WA\"\t53031\t\"San Juan County, WA\"\t53055\n\"King County, WA\"\t53033\t\"Chelan County, WA\"\t53007\n\"King County, WA\"\t53033\t\"King County, WA\"\t53033\n\"King County, WA\"\t53033\t\"Kitsap County, WA\"\t53035\n\"King County, WA\"\t53033\t\"Kittitas County, WA\"\t53037\n\"King County, WA\"\t53033\t\"Pierce County, WA\"\t53053\n\"King County, WA\"\t53033\t\"Snohomish County, WA\"\t53061\n\"King County, WA\"\t53033\t\"Yakima County, WA\"\t53077\n\"Kitsap County, WA\"\t53035\t\"Island County, WA\"\t53029\n\"Kitsap County, WA\"\t53035\t\"Jefferson County, WA\"\t53031\n\"Kitsap County, WA\"\t53035\t\"King County, WA\"\t53033\n\"Kitsap County, WA\"\t53035\t\"Kitsap County, WA\"\t53035\n\"Kitsap County, WA\"\t53035\t\"Mason County, WA\"\t53045\n\"Kitsap County, WA\"\t53035\t\"Pierce County, WA\"\t53053\n\"Kitsap County, WA\"\t53035\t\"Snohomish County, WA\"\t53061\n\"Kittitas County, WA\"\t53037\t\"Chelan County, WA\"\t53007\n\"Kittitas County, WA\"\t53037\t\"Douglas County, WA\"\t53017\n\"Kittitas County, WA\"\t53037\t\"Grant County, WA\"\t53025\n\"Kittitas County, WA\"\t53037\t\"King County, WA\"\t53033\n\"Kittitas County, WA\"\t53037\t\"Kittitas County, WA\"\t53037\n\"Kittitas County, WA\"\t53037\t\"Pierce County, WA\"\t53053\n\"Kittitas County, WA\"\t53037\t\"Yakima County, WA\"\t53077\n\"Klickitat County, WA\"\t53039\t\"Gilliam County, OR\"\t41021\n\"Klickitat County, WA\"\t53039\t\"Hood River County, OR\"\t41027\n\"Klickitat County, WA\"\t53039\t\"Morrow County, OR\"\t41049\n\"Klickitat County, WA\"\t53039\t\"Sherman County, OR\"\t41055\n\"Klickitat County, WA\"\t53039\t\"Wasco County, OR\"\t41065\n\"Klickitat County, WA\"\t53039\t\"Benton County, WA\"\t53005\n\"Klickitat County, WA\"\t53039\t\"Klickitat County, WA\"\t53039\n\"Klickitat County, WA\"\t53039\t\"Skamania County, WA\"\t53059\n\"Klickitat County, WA\"\t53039\t\"Yakima County, WA\"\t53077\n\"Lewis County, WA\"\t53041\t\"Cowlitz County, WA\"\t53015\n\"Lewis County, WA\"\t53041\t\"Grays Harbor County, WA\"\t53027\n\"Lewis County, WA\"\t53041\t\"Lewis County, WA\"\t53041\n\"Lewis County, WA\"\t53041\t\"Pacific County, WA\"\t53049\n\"Lewis County, WA\"\t53041\t\"Pierce County, WA\"\t53053\n\"Lewis County, WA\"\t53041\t\"Skamania County, WA\"\t53059\n\"Lewis County, WA\"\t53041\t\"Thurston County, WA\"\t53067\n\"Lewis County, WA\"\t53041\t\"Wahkiakum County, WA\"\t53069\n\"Lewis County, WA\"\t53041\t\"Yakima County, WA\"\t53077\n\"Lincoln County, WA\"\t53043\t\"Adams County, WA\"\t53001\n\"Lincoln County, WA\"\t53043\t\"Ferry County, WA\"\t53019\n\"Lincoln County, WA\"\t53043\t\"Grant County, WA\"\t53025\n\"Lincoln County, WA\"\t53043\t\"Lincoln County, WA\"\t53043\n\"Lincoln County, WA\"\t53043\t\"Okanogan County, WA\"\t53047\n\"Lincoln County, WA\"\t53043\t\"Spokane County, WA\"\t53063\n\"Lincoln County, WA\"\t53043\t\"Stevens County, WA\"\t53065\n\"Lincoln County, WA\"\t53043\t\"Whitman County, WA\"\t53075\n\"Mason County, WA\"\t53045\t\"Grays Harbor County, WA\"\t53027\n\"Mason County, WA\"\t53045\t\"Jefferson County, WA\"\t53031\n\"Mason County, WA\"\t53045\t\"Kitsap County, WA\"\t53035\n\"Mason County, WA\"\t53045\t\"Mason County, WA\"\t53045\n\"Mason County, WA\"\t53045\t\"Pierce County, WA\"\t53053\n\"Mason County, WA\"\t53045\t\"Thurston County, WA\"\t53067\n\"Okanogan County, WA\"\t53047\t\"Chelan County, WA\"\t53007\n\"Okanogan County, WA\"\t53047\t\"Douglas County, WA\"\t53017\n\"Okanogan County, WA\"\t53047\t\"Ferry County, WA\"\t53019\n\"Okanogan County, WA\"\t53047\t\"Grant County, WA\"\t53025\n\"Okanogan County, WA\"\t53047\t\"Lincoln County, WA\"\t53043\n\"Okanogan County, WA\"\t53047\t\"Okanogan County, WA\"\t53047\n\"Okanogan County, WA\"\t53047\t\"Skagit County, WA\"\t53057\n\"Okanogan County, WA\"\t53047\t\"Whatcom County, WA\"\t53073\n\"Pacific County, WA\"\t53049\t\"Clatsop County, OR\"\t41007\n\"Pacific County, WA\"\t53049\t\"Grays Harbor County, WA\"\t53027\n\"Pacific County, WA\"\t53049\t\"Lewis County, WA\"\t53041\n\"Pacific County, WA\"\t53049\t\"Pacific County, WA\"\t53049\n\"Pacific County, WA\"\t53049\t\"Wahkiakum County, WA\"\t53069\n\"Pend Oreille County, WA\"\t53051\t\"Bonner County, ID\"\t16017\n\"Pend Oreille County, WA\"\t53051\t\"Boundary County, ID\"\t16021\n\"Pend Oreille County, WA\"\t53051\t\"Pend Oreille County, WA\"\t53051\n\"Pend Oreille County, WA\"\t53051\t\"Spokane County, WA\"\t53063\n\"Pend Oreille County, WA\"\t53051\t\"Stevens County, WA\"\t53065\n\"Pierce County, WA\"\t53053\t\"King County, WA\"\t53033\n\"Pierce County, WA\"\t53053\t\"Kitsap County, WA\"\t53035\n\"Pierce County, WA\"\t53053\t\"Kittitas County, WA\"\t53037\n\"Pierce County, WA\"\t53053\t\"Lewis County, WA\"\t53041\n\"Pierce County, WA\"\t53053\t\"Mason County, WA\"\t53045\n\"Pierce County, WA\"\t53053\t\"Pierce County, WA\"\t53053\n\"Pierce County, WA\"\t53053\t\"Thurston County, WA\"\t53067\n\"Pierce County, WA\"\t53053\t\"Yakima County, WA\"\t53077\n\"San Juan County, WA\"\t53055\t\"Clallam County, WA\"\t53009\n\"San Juan County, WA\"\t53055\t\"Island County, WA\"\t53029\n\"San Juan County, WA\"\t53055\t\"Jefferson County, WA\"\t53031\n\"San Juan County, WA\"\t53055\t\"San Juan County, WA\"\t53055\n\"San Juan County, WA\"\t53055\t\"Skagit County, WA\"\t53057\n\"San Juan County, WA\"\t53055\t\"Whatcom County, WA\"\t53073\n\"Skagit County, WA\"\t53057\t\"Chelan County, WA\"\t53007\n\"Skagit County, WA\"\t53057\t\"Island County, WA\"\t53029\n\"Skagit County, WA\"\t53057\t\"Okanogan County, WA\"\t53047\n\"Skagit County, WA\"\t53057\t\"San Juan County, WA\"\t53055\n\"Skagit County, WA\"\t53057\t\"Skagit County, WA\"\t53057\n\"Skagit County, WA\"\t53057\t\"Snohomish County, WA\"\t53061\n\"Skagit County, WA\"\t53057\t\"Whatcom County, WA\"\t53073\n\"Skamania County, WA\"\t53059\t\"Hood River County, OR\"\t41027\n\"Skamania County, WA\"\t53059\t\"Multnomah County, OR\"\t41051\n\"Skamania County, WA\"\t53059\t\"Clark County, WA\"\t53011\n\"Skamania County, WA\"\t53059\t\"Cowlitz County, WA\"\t53015\n\"Skamania County, WA\"\t53059\t\"Klickitat County, WA\"\t53039\n\"Skamania County, WA\"\t53059\t\"Lewis County, WA\"\t53041\n\"Skamania County, WA\"\t53059\t\"Skamania County, WA\"\t53059\n\"Skamania County, WA\"\t53059\t\"Yakima County, WA\"\t53077\n\"Snohomish County, WA\"\t53061\t\"Chelan County, WA\"\t53007\n\"Snohomish County, WA\"\t53061\t\"Island County, WA\"\t53029\n\"Snohomish County, WA\"\t53061\t\"King County, WA\"\t53033\n\"Snohomish County, WA\"\t53061\t\"Kitsap County, WA\"\t53035\n\"Snohomish County, WA\"\t53061\t\"Skagit County, WA\"\t53057\n\"Snohomish County, WA\"\t53061\t\"Snohomish County, WA\"\t53061\n\"Spokane County, WA\"\t53063\t\"Benewah County, ID\"\t16009\n\"Spokane County, WA\"\t53063\t\"Bonner County, ID\"\t16017\n\"Spokane County, WA\"\t53063\t\"Kootenai County, ID\"\t16055\n\"Spokane County, WA\"\t53063\t\"Lincoln County, WA\"\t53043\n\"Spokane County, WA\"\t53063\t\"Pend Oreille County, WA\"\t53051\n\"Spokane County, WA\"\t53063\t\"Spokane County, WA\"\t53063\n\"Spokane County, WA\"\t53063\t\"Stevens County, WA\"\t53065\n\"Spokane County, WA\"\t53063\t\"Whitman County, WA\"\t53075\n\"Stevens County, WA\"\t53065\t\"Ferry County, WA\"\t53019\n\"Stevens County, WA\"\t53065\t\"Lincoln County, WA\"\t53043\n\"Stevens County, WA\"\t53065\t\"Pend Oreille County, WA\"\t53051\n\"Stevens County, WA\"\t53065\t\"Spokane County, WA\"\t53063\n\"Stevens County, WA\"\t53065\t\"Stevens County, WA\"\t53065\n\"Thurston County, WA\"\t53067\t\"Grays Harbor County, WA\"\t53027\n\"Thurston County, WA\"\t53067\t\"Lewis County, WA\"\t53041\n\"Thurston County, WA\"\t53067\t\"Mason County, WA\"\t53045\n\"Thurston County, WA\"\t53067\t\"Pierce County, WA\"\t53053\n\"Thurston County, WA\"\t53067\t\"Thurston County, WA\"\t53067\n\"Wahkiakum County, WA\"\t53069\t\"Clatsop County, OR\"\t41007\n\"Wahkiakum County, WA\"\t53069\t\"Columbia County, OR\"\t41009\n\"Wahkiakum County, WA\"\t53069\t\"Cowlitz County, WA\"\t53015\n\"Wahkiakum County, WA\"\t53069\t\"Lewis County, WA\"\t53041\n\"Wahkiakum County, WA\"\t53069\t\"Pacific County, WA\"\t53049\n\"Wahkiakum County, WA\"\t53069\t\"Wahkiakum County, WA\"\t53069\n\"Walla Walla County, WA\"\t53071\t\"Umatilla County, OR\"\t41059\n\"Walla Walla County, WA\"\t53071\t\"Benton County, WA\"\t53005\n\"Walla Walla County, WA\"\t53071\t\"Columbia County, WA\"\t53013\n\"Walla Walla County, WA\"\t53071\t\"Franklin County, WA\"\t53021\n\"Walla Walla County, WA\"\t53071\t\"Walla Walla County, WA\"\t53071\n\"Whatcom County, WA\"\t53073\t\"Okanogan County, WA\"\t53047\n\"Whatcom County, WA\"\t53073\t\"San Juan County, WA\"\t53055\n\"Whatcom County, WA\"\t53073\t\"Skagit County, WA\"\t53057\n\"Whatcom County, WA\"\t53073\t\"Whatcom County, WA\"\t53073\n\"Whitman County, WA\"\t53075\t\"Benewah County, ID\"\t16009\n\"Whitman County, WA\"\t53075\t\"Latah County, ID\"\t16057\n\"Whitman County, 
